vi "Test Stop.vi"(11 "Error in":errorcluster) -> (15 "Error out":errorcluster)   [LabVIEW 2020, in "StopWatchTests.lvlib"]
doc: "This VI validates the stop button"
uses:
  <vilib>/SLL Drona/APIs/Assert/AssertVI/AssertVIExecRunning.vi
  <vilib>/SLL Drona/APIs/Stimulus/ControlValue/SetValueAuto.vi
  <vilib>/SLL Drona/APIs/Assert/AssertVI/AssertVIExecIdle.vi
  <vilib>/SLL Drona/APIs/Stimulus/VI/CloseVI.vi
  StopWatchTests.lvlib
  <vilib>/SLL Drona/Drona.lvlib
  <vilib>/addons/_JKI Toolkits/Caraya/classes/Test/Test.lvclass
  <vilib>/SLL Drona/APIs/Assert/AssertVI/AssertVI.lvlib
  <vilib>/SLL Drona/APIs/Stimulus/ControlValue/ControlValue.lvlib
  <vilib>/SLL Drona/APIs/Stimulus/VI/VI.lvlib
panel:
  # "STOP TEST"
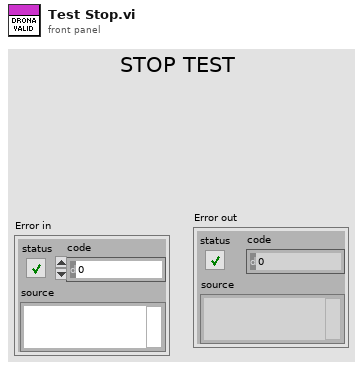
[diagram p1: front panel]
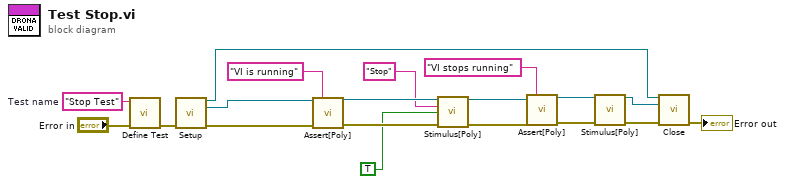
[diagram p0: block diagram]
diagram:
  w17 = "Stop Test"  # Test name
  n1 = call <vilib>:"Define Test.vi"("error in (no error)"="Error in", "Label (VI Title)"=w17) -> ("error out"=w18:errorcluster)  [unwired: 9 in]
  n2 = call <vilib>:"Setup.vi"("error in"=w18) -> ("Application Ref"=w16:refnum<vi>, "VI Reference Out"=w10:refnum<vi>, "error out"=w12:errorcluster)  [unwired: 12 in]
  n3 = call-poly <vilib>:"Assert[Poly].vi"("VI Reference In"=w10, "Test Label"="VI is running", "Error In"=w12) -> ("VI Reference Out"=w8:refnum<vi>, "Error Out"=w9:errorcluster)  [unwired: 11 in]
  n4 = call-poly <vilib>:"Stimulus[Poly].vi"("VI Reference In"=w8, "Control Path"="Stop", "Value (Signaling)"=TRUE, "error in"=w9) -> ("VI Reference Out"=w4:refnum<vi>, "error out"=w5:errorcluster)  [unwired: 10 in]
  n5 = call-poly <vilib>:"Assert[Poly].vi"("VI Reference In"=w4, "Test Label"="VI stops running", "Error In"=w5) -> ("VI Reference Out"=w1:refnum<vi>, "Error Out"=w2:errorcluster)  [unwired: 11 in]
  n6 = call-poly <vilib>:"Stimulus[Poly].vi"("VI Reference In"=w1, "error in"=w2) -> ("VI Reference Out"=w15:refnum<vi>, "error out"=w14:errorcluster)  [unwired: 12 in]
  n7 = call <vilib>:"Close.vi"("Application Ref"=w16, "VI Reference"=w15, "error in"=w14) -> ("error out"=→"Error out":errorcluster)  [unwired: 12 in]
